vi "BME_DG_ReadCalibrConst_from_File.vi"(8 "error in (no error)":errorcluster, 11 "Path":path) -> (0 "error out":errorcluster, 3 "return code":i32)   [LabVIEW 2009, in "POLARIS BME DG.lvlib"]
uses:
  POLARIS BME DG.lvlib
  BME DLL/DelayGenerator.dll
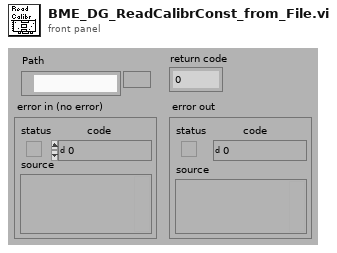
[diagram p1: front panel]
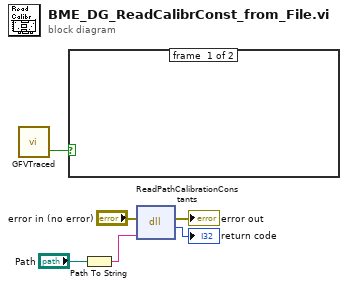
[diagram p0: block diagram]
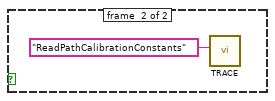
[diagram p2: hidden frame]
diagram:
  n1 = call "GFVTraced.vi"() -> ("traced?"=w1:bool)  [unwired: 2 in]
  n2 = case shown="True" w1 {
    frame #0 {
    }
    frame #1 {
      n3 = call "TRACE.vi"("Function"="ReadPathCalibrationConstants") -> ()  [unwired: 11 in]
    }
  }
  n4 = Path To String(path="Path") -> (string=w2:string)
  n5 = dll-call lib="D:/CS Framework/LVSCC/LV2009/GPL/Projects/cs-framework/CSClass/CSPOLARIS/POLARIS BME DG/BME DLL/DelayGenerator.dll" fn="ReadPathCalibrationConstants"(error in="error in (no error)", "Path"=w2) -> (error out=→"error out":errorcluster, "return type"=→"return code":i32)  [unwired: 3 in, 1 out]
